vi "BooleanOperators.vi"() -> ()   [LabVIEW 2020]
panel:
  out "XOR":bool
  out "NOR":bool
  out "NAND":bool
  out "OR":bool
  out "AND":bool
  in  "B":bool
  in  "A":bool
  # "Boolean Opeartors"
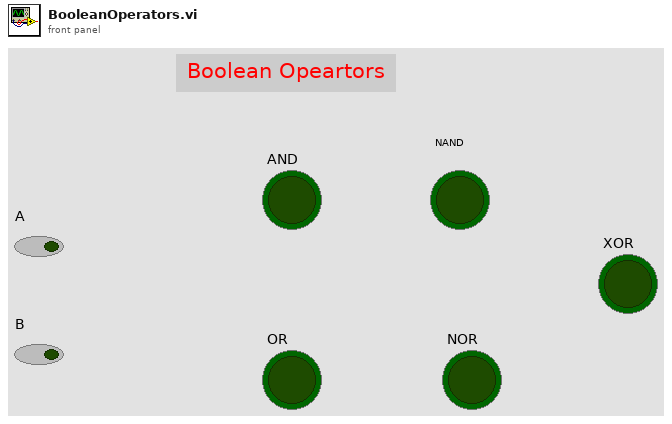
[diagram p1: front panel]
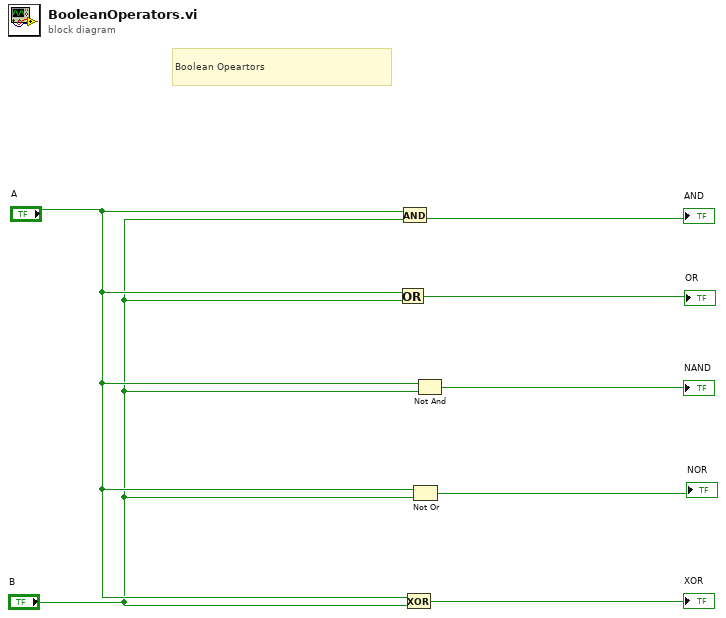
[diagram p0: block diagram]
diagram:
  # "Boolean Opeartors"
  n1 = Or(x="A", y="B") -> (x .or. y?=→"OR":bool)
  n2 = And(x="A", y="B") -> (x .and. y?=→"AND":bool)
  n3 = Exclusive Or(1:"B", 2:"A") -> (0:→"XOR":bool)
  n4 = Not Or(1:"B", 2:"A") -> (0:→"NOR":bool)
  n5 = Not And(1:"B", 2:"A") -> (0:→"NAND":bool)
